vi "init VIs.vi"(8 "error in (no error)":errorcluster, 11 "S4GEI in":refnum<class "S4GEI.lvclass">) -> (0 "error out":errorcluster, 3 "S4GEI out":refnum<class "S4GEI.lvclass">)   [LabVIEW 2018, in "S4GEI.lvclass"]
uses:
  S4GEI.lvclass
  S4GEI.lvclass/S4GEI.ctl
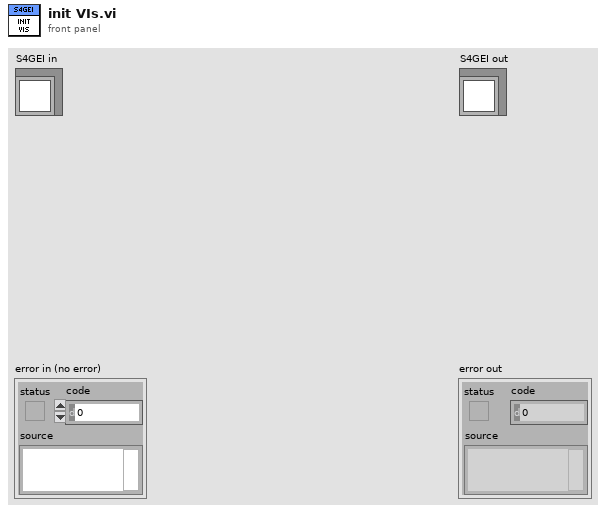
[diagram p1: front panel]
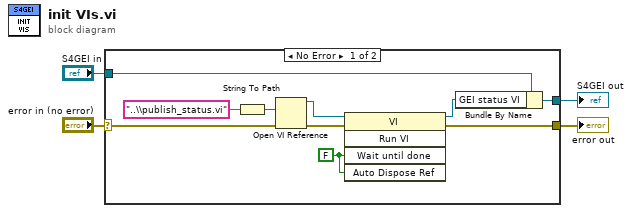
[diagram p0: block diagram]
diagram:
  n1 = case shown="No Error" "error in (no error)" {
    selector: "error in (no error)" -> [w10 w16]
    tunnel: [w9 w16] -> w3
    tunnel: [w6 w15] -> w1
    tunnel: "S4GEI in" -> [w7 w15]
    frame No Error {
      w13 = FALSE ("Wait Until Done")
      n2 = String To Path(string="..\\publish_status.vi" ("name or relative path")) -> (path=w11:path)
      n3 = Open VI Reference(vi path=w11, error in (no error)=w10) -> (vi reference=w14:refnum<vi>, error out=w12:errorcluster)  [unwired: 4 in]
      n4 = invoke class="VI" method="Run VI"(reference=w14, error in=w12, "Wait until done"=w13, "Auto Dispose Ref"=w13) -> (reference out=w5:refnum<vi>, error out=w9:errorcluster)  [unwired: 1 in, 3 out]
      n5 = Bundle By Name(cluster=w7, "GEI status VI"=w5) -> (w6:refnum<class "S4GEI.lvclass">)
    }
    frame Error {
    }
  }
  "error out" <- w3
  "S4GEI out" <- w1
